vi "GPS -MIN Distance from Point.vi"(0 "POI-Lat":dbl, 2 "POI-Lng":dbl, 3 "arrLatLng|ID":string[][](array[string]), 5 "error in (no error)":errorcluster) -> (14 "DataArry -OUT":string[][](array[string]), 19 "error out":errorcluster)   [LabVIEW 2019]
uses:
  ctlGPSColIdxs.ctl
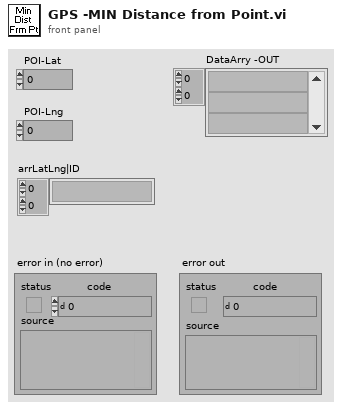
[diagram p1: front panel]
types:
  T1 = typedef "ctlGPSColIdxs.ctl" = enum16{"#", "Vw", "Year", "Project Info", "Address", "Lat", "Lng", "Icon -Maps", "Icon -Custom", "EIDProj", "EIDAddr", "OnMap"}
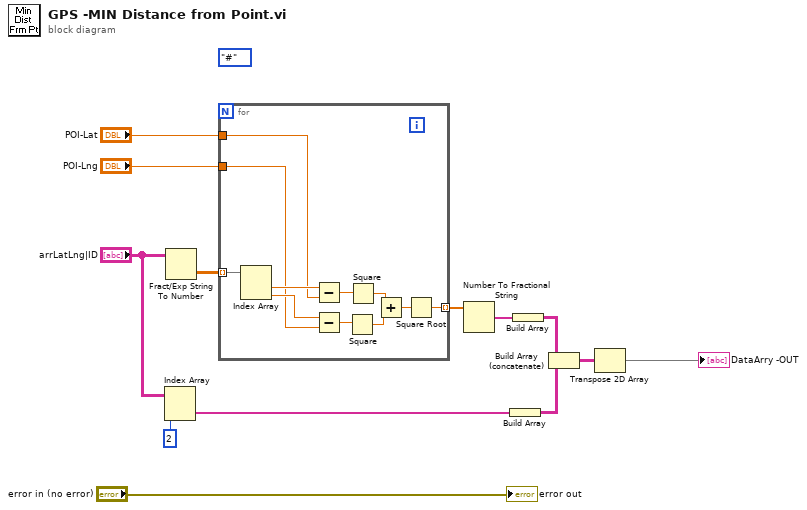
[diagram p0: block diagram]
diagram:
  (unwired) ctlGPSColIdxs."#" ("ColIdxs")
  n1 = Index Array(array="arrLatLng|ID", index (col)=2 ("disabled index (col)")) -> (element=w6:string[])  [unwired: 1 in]
  n2 = Fract/Exp String To Number(string="arrLatLng|ID") -> (number=w11:dbl[][])  [unwired: 3 in, 1 out]
  n3 = for {
    tunnel: "POI-Lat" -> [w22]
    tunnel: "POI-Lng" -> [w20]
    tunnel: w11 -> [w24] mode=indexing
    tunnel: [w14] -> w10 mode=indexing
    n4 = Index Array(array=w24) -> (element #1=w23:dbl, element #2=w21:dbl)  [unwired: 2 in]
    n5 = Subtract(x=w23, y=w22) -> (x-y=w19:dbl)
    n6 = Subtract(x=w21, y=w20) -> (x-y=w18:dbl)
    n7 = Square(x=w18) -> (x^2=w17:dbl)
    n8 = Square(x=w19) -> (x^2=w16:dbl)
    n9 = Add(x=w16, y=w17) -> (x+y=w15:dbl)
    n10 = Square Root(x=w15) -> (sqrt(x)=w14:dbl)
  }
  n11 = Number To Fractional String(number=w10) -> (F-format string=w9:string[])  [unwired: 3 in]
  n12 = Build Array(w6) -> (w4:string[][])
  n13 = Build Array(w9) -> (w5:string[][])
  n14 = Build Array (concatenate)(w5, w4) -> (w3:string[][])
  n15 = Transpose 2D Array(2D array=w3) -> (transposed array=→"DataArry -OUT":string[][])
  "error out" <- "error in (no error)"
